vi "Write From DRAM Ref.vi"(10 "From DRAM":refnum<k21>, 11 "K7 DRAM FIFO in":refnum<class "K7 DRAM FIFO.lvclass">) -> (3 "K7 DRAM FIFO out":refnum<class "K7 DRAM FIFO.lvclass">)   [LabVIEW 2015, in "K7 DRAM FIFO.lvclass"]
uses:
  K7 DRAM FIFO.lvclass
  K7 DRAM FIFO.lvclass/K7 DRAM FIFO.ctl
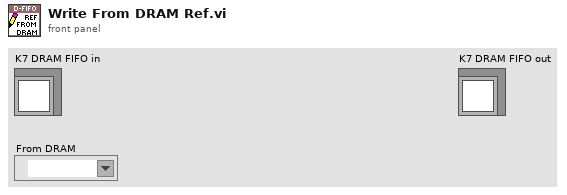
[diagram p1: front panel]
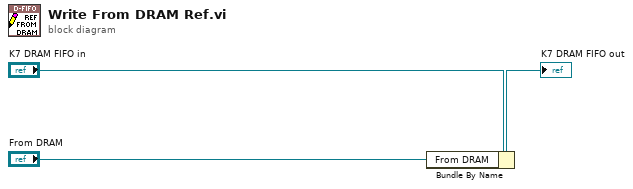
[diagram p0: block diagram]
diagram:
  n1 = Bundle By Name(cluster="K7 DRAM FIFO in", "From DRAM"="From DRAM") -> (→"K7 DRAM FIFO out":refnum<class "K7 DRAM FIFO.lvclass">)
